vi "GenerateHarmonicArray.vi"(1 "Samples":dbl[](array[numeric]) format="%.2f", 2 "Harmonic":u8, 3 "input":dbl format="%.2f") -> (0 "Ouput Samples":dbl[](array[numeric]) format="%.2f")   [LabVIEW 2021]
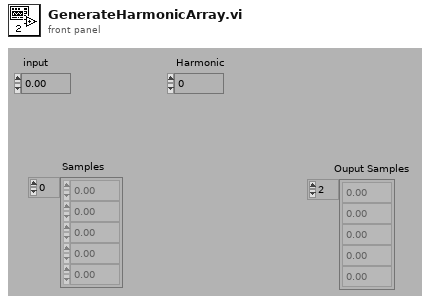
[diagram p1: front panel]
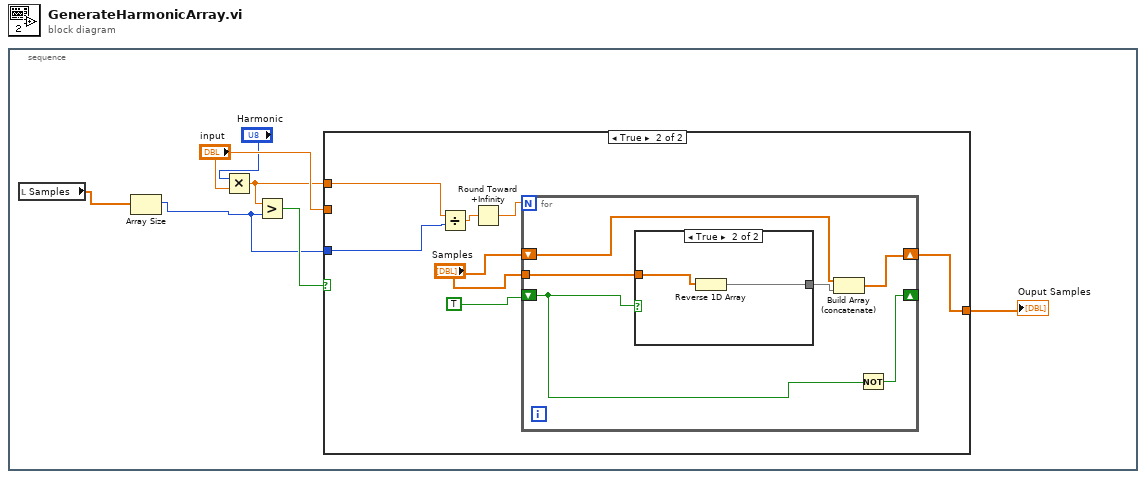
[diagram p0: block diagram]
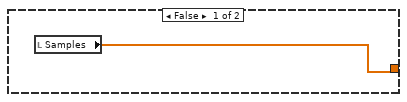
[diagram p2: hidden frame]
diagram:
  n1 = stacked-sequence {
    frame #0 {
      n2 = local read "Samples"() -> (w2:dbl[])
      n3 = Array Size(array=w2) -> (size(s)=w1:i32)
      n4 = Multiply(x="Harmonic", y="input") -> (x*y=w3:dbl)
      n5 = Greater?(x=w3, y=w1) -> (0:w7:bool)
      n6 = case shown="True" w7 {
        tunnel: "input" -> [_ _]
        tunnel: w1 -> [_ w11]
        tunnel: [w8 w13] -> w6
        tunnel: w3 -> [_ w12]
        frame False {
          n7 = local read "Samples"() -> (w8:dbl[])
        }
        frame True {
          n8 = Divide(x=w12, y=w11) -> (x/y=w10:dbl)
          n9 = Round Toward +Infinity(x=w10) -> (ceil(x): smallest int >= x=w9:dbl)
          n10 = for {
            N: w9 -> [_]
            shift-right: [w21] -> _
            shift-left: TRUE -> [w20]
            shift-right: [w16] -> w13
            shift-left: "Samples" -> [w18]
            tunnel: "Samples" -> [w19]
            n11 = case shown="True" w20 {
              tunnel: w19 -> [w22 w24]
              tunnel: [w22 w23] -> w17
              frame False {
              }
              frame True {
                n12 = Reverse 1D Array(array=w24) -> (reversed array=w23:dbl[])
              }
            }
            n13 = Build Array (concatenate)(w18, w17) -> (w16:dbl[])
            n14 = Not(x=w20) -> (.not. x?=w21:bool)
          }
        }
      }
      "Ouput Samples" <- w6
    }
  }
